vi "Video Playback Using Javascript.vi"() -> ()   [LabVIEW 2026]
doc: "Uses a Web Browser to play an instructional video, and programmatically respond as play progresses using Javascript."
panel:
  out "Web Browser Control":string(html)="about:blank"
  out "JS Message":string
  in  "Stop":bool
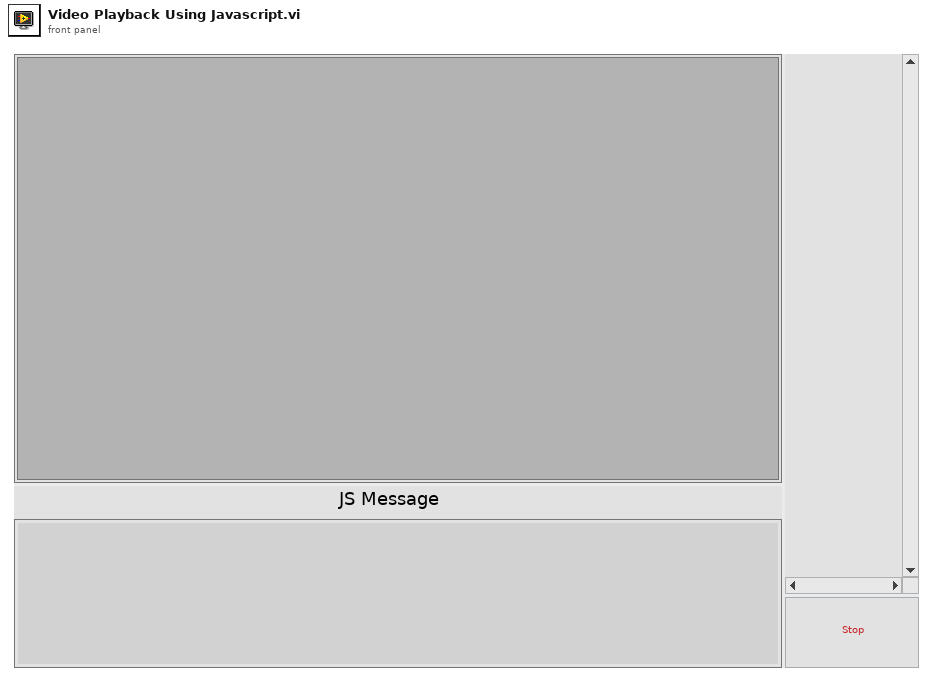
[diagram p1: front panel]
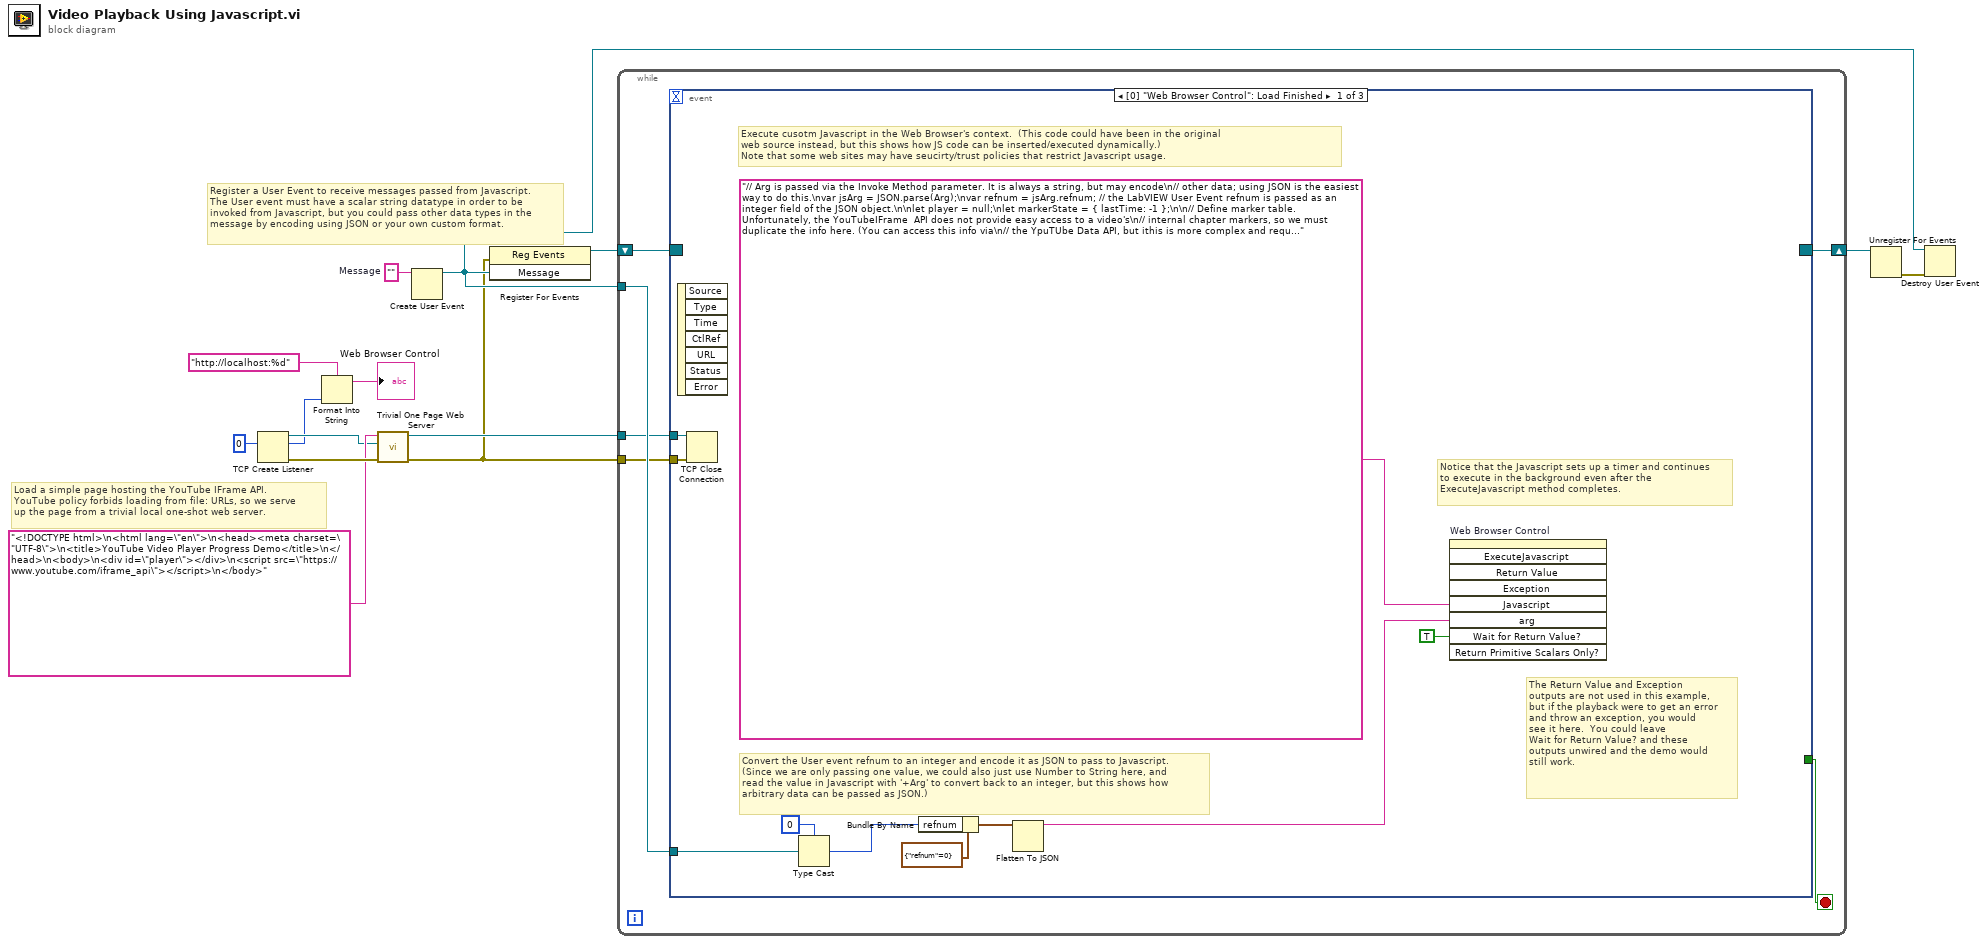
[diagram p0: block diagram]
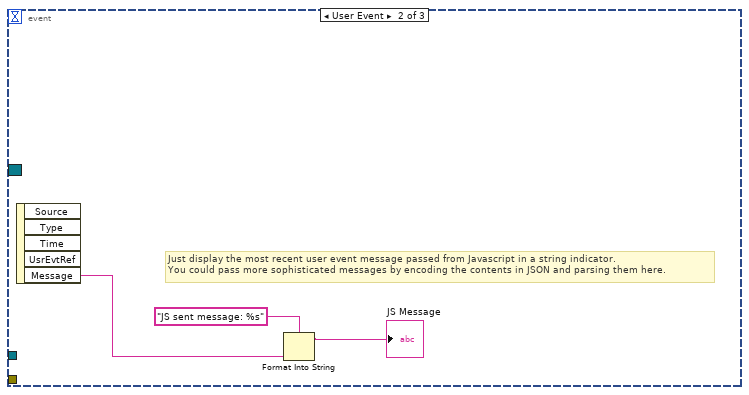
[diagram p2: hidden frame]
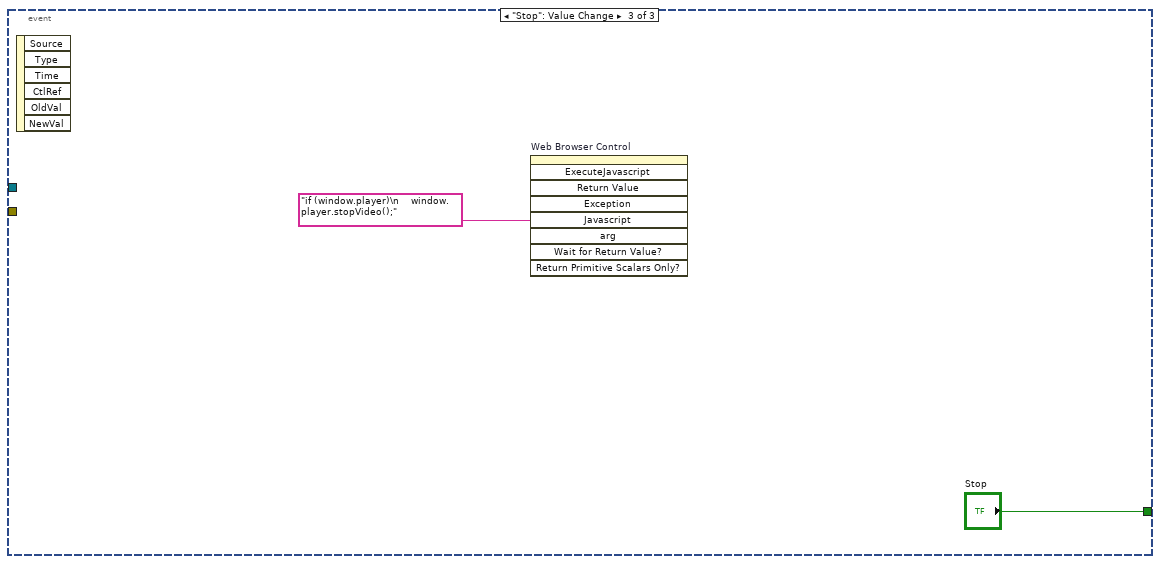
[diagram p3: hidden frame]
diagram:
  w14 = ""  # Message
  # "Load a simple page hosting the YouTube IFrame API.\nYouTube policy forbids loading from file: URLs, so we serve\nup the page from a trivial local one-shot web server."
  # "Register a User Event to receive messages passed from Javascript.\nThe User event must have a scalar string datatype in order to be\ninvoked from Javascript, but you could pass other data types in the\nmessage by encoding using JSON or your own custom format."
  n1 = TCP Create Listener(10:u16 0 ("port")) -> (0:w10:errorcluster, 2:w3:u16, 3:w5:refnum<k5>)  [unwired: 4 in]
  n2 = Format Into String(format string="http://localhost:%d", w3) -> (resulting string=→"Web Browser Control":string)  [unwired: 2 in, 1 out]
  n3 = call "Trivial One Page Web Server.vi"("error in"=w10, "listener ID in"=w5, "HTML Content"="<!DOCTYPE html>\n<html lang=\"en\">\n<head><meta charset=\"UTF-8\">\n<title>YouTube Video Player Progress Demo</title>\n</head>\n<body>\n<div id=\"player\"></div>\n<script src=\"https://www.youtube.com/iframe_api\"></script>\n</body>") -> ("error out"=w1:errorcluster, "connection ID out"=w2:refnum<k5>)  [unwired: 7 in]
  n4 = Create User Event(user event datatype=w14) -> (user event=w7:refnum<user-event>)  [unwired: 1 in, 1 out]
  n5 = register-events(error in=w1, w7) -> (reference out=w13:refnum<event-registration>)  [unwired: 1 in, 1 out]
  n6 = while {
    tunnel: w7 -> [w18]
    shift-right: [w17] -> w8
    shift-left: w13 -> [w19]
    tunnel: w2 -> [w16]
    tunnel: w1 -> [w15]
    stop <- w20 stop-if-true
    n7 = event shown="[0] \"Web Browser Control\": Load Finished" {
      selector: w19 -> [_ _ _]
      dyn-events: [_ _ _] -> w17
      timeout: _ -> [_ _ _]
      tunnel: [_ _ "Stop"] -> w20
      tunnel: w18 -> [w30 _ _]
      tunnel: w16 -> [w29 _ _]
      tunnel: w15 -> [w28 _ _]
      event "Web Browser Control": Load Finished {
        # "Notice that the Javascript sets up a timer and continues\nto execute in the background even after the\nExecuteJavascript method completes."
        # "The Return Value and Exception\noutputs are not used in this example,\nbut if the playback were to get an error \nand throw an exception, you would\nsee it here.  You could leave\nWait for Return Value? and these\noutputs unwired and the demo would\nstill work."
        # "Convert the User event refnum to an integer and encode it as JSON to pass to Javascript.\n(Since we are only passing one value, we could also just use Number to String here, and\nread the value in Javascript with '+Arg' to convert back to an integer, but this shows how\narbitrary data can be passed as JSON.)"
        # "Execute cusotm Javascript in the Web Browser's context.  (This code could have been in the original\nweb source instead, but this shows how JS code can be inserted/executed dynamically.)\nNote that some web sites may have seucirty/trust policies that restrict Javascript usage."
        n8 = event-data() -> ()  [unwired: 1 in, 7 out]
        n9 = TCP Close Connection(connection ID=w29, error in (no error)=w28) -> ()  [unwired: 1 in, 2 out]
        n10 = Type Cast(type=u32 0, x=w30) -> (*(type *) &x=w24:u32)
        n11 = Bundle By Name(cluster=cluster{"refnum":u32} {"refnum"=0}, "refnum"=w24) -> (w26:cluster{"refnum":u32})
        n12 = Flatten To JSON(anything=w26) -> (JSON string=w22:string)  [unwired: 2 in, 1 out]
        n13 = invoke on="Web Browser Control" class="WebBrowser (strict)" method="ExecuteJavascript"("Javascript"="// Arg is passed via the Invoke Method parameter. It is always a string, but may encode\n// other data; using JSON is the easiest way to do this.\nvar jsArg = JSON.parse(Arg);\nvar refnum = jsArg.refnum; // the LabVIEW User Event refnum is passed as an integer field of the JSON object.\n\nlet player = null;\nlet markerState = { lastTime: -1 };\n\n// Define marker table.  Unfortunately, the YouTubeIFrame  API does not provide easy access to a video's\n// internal chapter markers, so we must duplicate the info here. (You can access this info via\n// the YpuTUbe Data API, but ithis is more complex and requires an API key.)\nconst markers = [\n    { time: 0,   message: \"Playing Introduction\" },\n    { time: 13,  message: \"LabVIEW Interface\" },\n    { time: 34, message: \"Controls palette\" },\n    { time: 112,  message: \"String palette\" },\n    { time: 149,  message: \"String constant\" },\n    { time: 161,  message: \"Hello world!\" },\n    { time: 174,  message: \"Run\" },\n];\n\n// Pass a message to LabVIEW via a User event\nfunction notify(message) {\n    // The event will be handled by another case of the Event structure.\n    LabVIEW.FireUserEvent(refnum, message);\n}\n\n// Called when the YouTube player has finished initializing\nfunction onPlayerReady(event) {\n    // Stash the player in the global window object, so the 'Stop' event can stop the video;\n    // (ExecuteJavascript code executes in an anonymous function scope, so variables are\n    // not visible in other instances, but you can add them to existing global JS objects such\n    // as window in order to persist them between instances.)\n    window.player = player; \n\n    setInterval(() => {\n        if (!player || player.getPlayerState() !== YT.PlayerState.PLAYING)\n            return;\n\n        const now = player.getCurrentTime();\n        const last = markerState.lastTime;\n\n        // Check for crossed markers\n        for (const m of markers) {\n            if (last < m.time && now >= m.time) {\n                notify(m.message);\n            }\n        }\n        markerState.lastTime = now;\n    }, 100); // Polling interval (100ms)\n}\n\n// If this code was in the original referring web page, this function would be called automatically\n// by the IFrame API. \nfunction onYouTubeIframeAPIReady() {\n    player = new YT.Player('player', {\n        width: 640,\n        height: 360,\n        videoId: \"ZHNlKyYzrPE\",\n        playerVars: { // mute is needed because YT prevents programmatic autoplay of non-muted videos\n            rel: 0, autoplay : 1, mute: 1, playsinline: 1\n        },\n        events: {\n            'onReady': onPlayerReady\n        }\n    });\n}\n// Running this code in the Web Browser control's 'Load Finished' method also ensures\n// the API is ready, so we call the function directly.\nonYouTubeIframeAPIReady();\nreturn 0;" ("Javascript String"), "arg"=w22, "Wait for Return Value?"=TRUE) -> ()  [unwired: 6 in, 9 out]
      }
      event User Event {
        # "Just display the most recent user event message passed from Javascript in a string indicator.\nYou could pass more sophisticated messages by encoding the contents in JSON and parsing them here."
        n14 = event-data() -> ("Message"=w32:string)  [unwired: 1 in, 4 out]
        n15 = Format Into String(format string="JS sent message: %s" ("message"), w32) -> (resulting string=→"JS Message":string)  [unwired: 2 in, 1 out]
      }
      event "Stop": Value Change {
        n16 = event-data() -> ()  [unwired: 1 in, 6 out]
        n17 = invoke on="Web Browser Control" class="WebBrowser (strict)" method="ExecuteJavascript"("Javascript"="if (window.player)\n    window.player.stopVideo();" ("Javascript String")) -> ()  [unwired: 8 in, 9 out]
      }
    }
  }
  n18 = Unregister For Events(event registration refnum=w8) -> (error out=w6:errorcluster)  [unwired: 1 in]
  n19 = Destroy User Event(user event=w7, error in=w6) -> ()  [unwired: 1 out]
